vi "Untitled 1.vi"() -> ()   [LabVIEW 2023]
panel:
  out "concatenated string":string
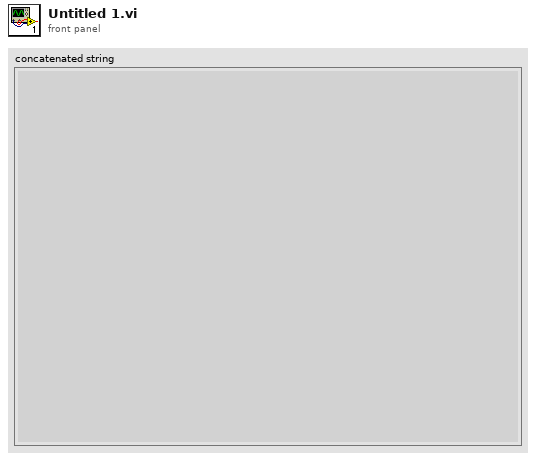
[diagram p1: front panel]
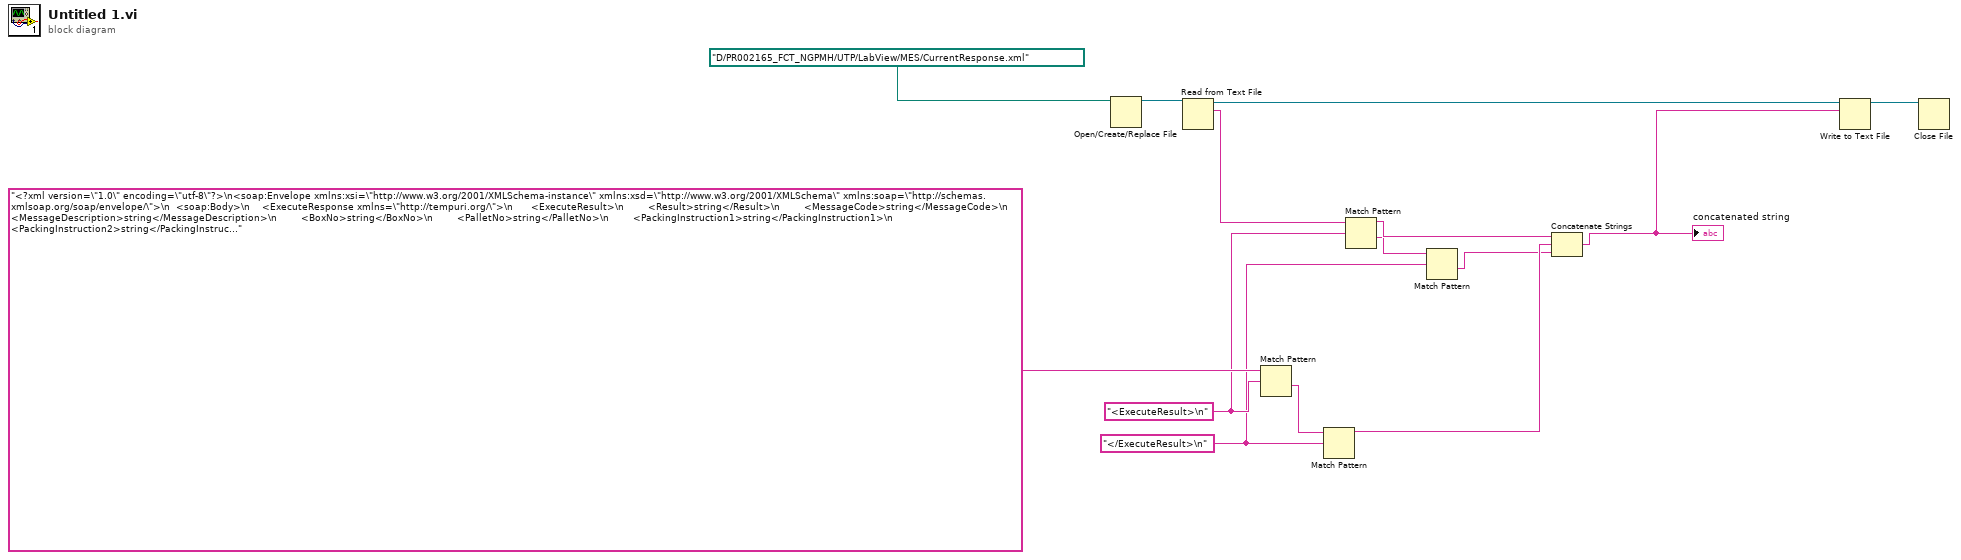
[diagram p0: block diagram]
diagram:
  w7 = "</ExecuteResult>\n" ("regular expression")
  w8 = "<ExecuteResult>\n" ("regular expression")
  n1 = Open/Create/Replace File(file path (use dialog)=path "D:/PR002165_FCT_NGPMH/UTP/LabView/MES/CurrentResponse.xml") -> (refnum out=w13:refnum<file>)  [unwired: 5 in, 2 out]
  n2 = Read from Text File(file (use dialog)=w13) -> (refnum out=w3:refnum<file>, text=w11:string)  [unwired: 3 in, 2 out]
  n3 = Match Pattern(string="<?xml version=\"1.0\" encoding=\"utf-8\"?>\n<soap:Envelope xmlns:xsi=\"http://www.w3.org/2001/XMLSchema-instance\" xmlns:xsd=\"http://www.w3.org/2001/XMLSchema\" xmlns:soap=\"http://schemas.xmlsoap.org/soap/envelope/\">\n  <soap:Body>\n    <ExecuteResponse xmlns=\"http://tempuri.org/\">\n      <ExecuteResult>\n        <Result>string</Result>\n        <MessageCode>string</MessageCode>\n        <MessageDescription>string</MessageDescription>\n        <BoxNo>string</BoxNo>\n        <PalletNo>string</PalletNo>\n        <PackingInstruction1>string</PackingInstruction1>\n        <PackingInstruction2>string</PackingInstruction2>\n        <PackingInstruction3>string</PackingInstruction3>\n        <PackingInstruction4>string</PackingInstruction4>\n        <PackingInstruction5>string</PackingInstruction5>\n        <SerialCount>int</SerialCount>\n        <MaxSerialCount>int</MaxSerialCount>\n        <BoxCount>int</BoxCount>\n        <MaxBoxCount>int</MaxBoxCount>\n      </ExecuteResult>\n    </ExecuteResponse>\n  </soap:Body>\n</soap:Envelope>\n", regular expression=w8) -> (after substring=w9:string)  [unwired: 1 in, 3 out]
  n4 = Match Pattern(string=w9, regular expression=w7) -> (before substring=w5:string)  [unwired: 1 in, 3 out]
  n5 = Match Pattern(string=w11, regular expression=w8) -> (before substring=w6:string, after substring=w1:string)  [unwired: 1 in, 2 out]
  n6 = Match Pattern(string=w1, regular expression=w7) -> (after substring=w4:string)  [unwired: 1 in, 3 out]
  n7 = Concatenate Strings(w6, w5, w4) -> (w2:string)
  "concatenated string" <- w2
  n8 = Write to Text File(file (use dialog)=w3, text=w2) -> (refnum out=w12:refnum<file>)  [unwired: 2 in, 2 out]
  n9 = Close File(refnum=w12) -> ()  [unwired: 1 in, 2 out]
